vi "题目二.vi"() -> ()   [LabVIEW 2017]
panel:
  out "数字波形图":digitalwaveform(graph)
  in  "Digital Waveform":digitalwaveform(waveform)={"t0"=timestamp(0 s since 1904-01-01), "dt"=1.0, "Y"={"transitions"=[], "data"=[]}} caption="数字波形"
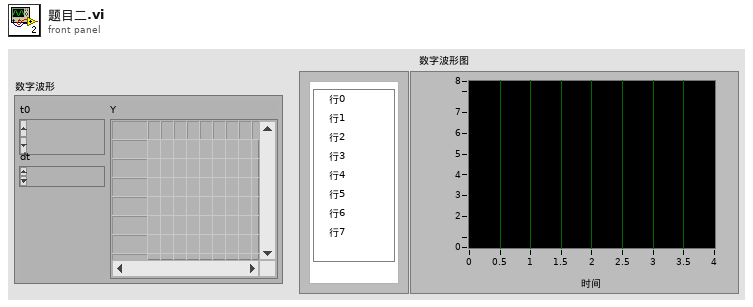
[diagram p1: front panel]
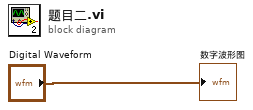
[diagram p0: block diagram]
diagram:
  "数字波形图" <- "Digital Waveform"
